vi "retrieveGoalAmount.vi"(8 "error in (no error)":errorcluster, 10 "Goal.lvclass":refnum<class "Goal.lvclass">, 11 "Account History in":refnum<class "Account History.lvclass">) -> (0 "error out":errorcluster, 2 "Amount":dbl, 3 "Account History out":refnum<class "Account History.lvclass">)   [LabVIEW 2018]
uses:
  Account History.lvclass
  Goal/Goal.lvclass
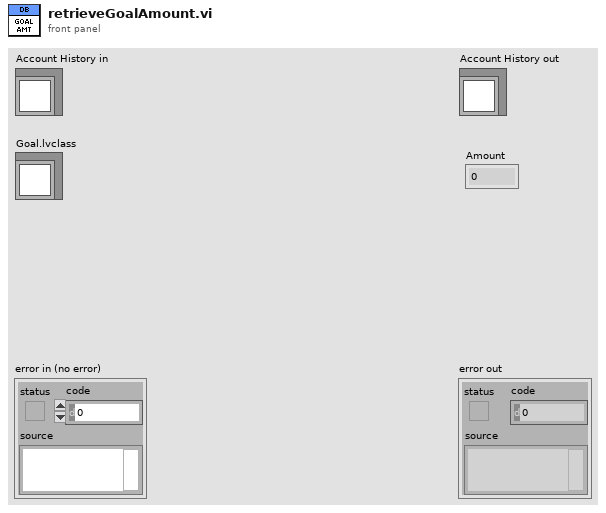
[diagram p1: front panel]
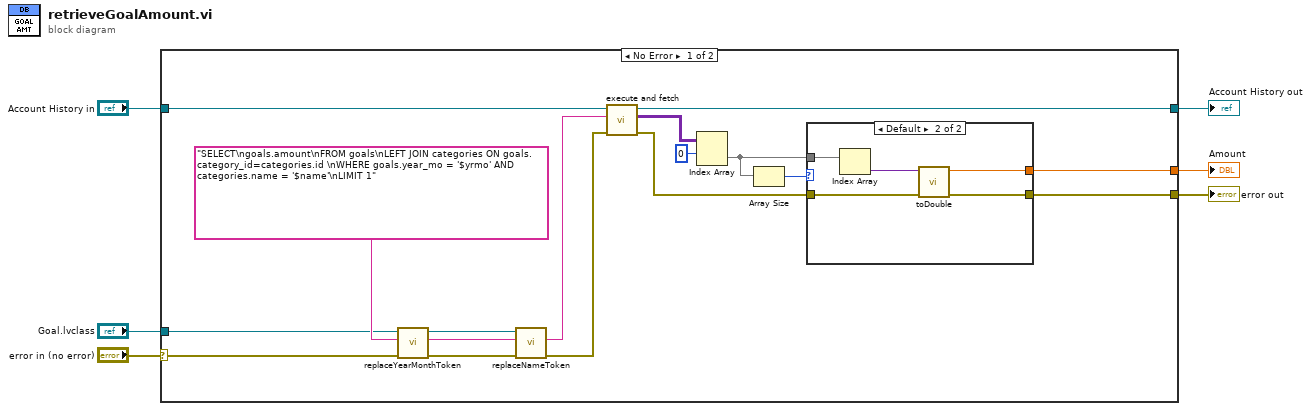
[diagram p0: block diagram]
diagram:
  n1 = case shown="No Error" "error in (no error)" {
    selector: "error in (no error)" -> [w17 w31]
    tunnel: [w21 w31] -> w5
    tunnel: [w22 w30] -> w3
    tunnel: "Account History in" -> [w23 w30]
    tunnel: "Goal.lvclass" -> [w12 _]
    tunnel: [w7 _] -> w1
    frame No Error {
      n2 = call "replaceYearMonthToken.vi"("error in (no error)"=w17, "Querry In"="SELECT\ngoals.amount\nFROM goals\nLEFT JOIN categories ON goals.category_id=categories.id \nWHERE goals.year_mo = '$yrmo' AND categories.name = '$name'\nLIMIT 1", "Goal in"=w12) -> ("error out"=w16:errorcluster, "Query Out"=w14:string, "Goal out"=w13:refnum<class "Goal.lvclass">)  [unwired: 6 in]
      n3 = call "replaceNameToken.vi"("error in (no error)"=w16, "Query In"=w14, "Goal in"=w13) -> ("error out"=w18:errorcluster, "Query Out"=w19:string)  [unwired: 6 in, 1 out]
      n4 = call "execute and fetch.vi"("error in (no error)"=w18, "SQL query"=w19, "Database in"=w23) -> ("error out"=w20:errorcluster, "recordset data"=w10:variant[][], "Database out"=w22:refnum<class "Account History.lvclass">)  [unwired: 5 in, 1 out]
      n5 = Index Array(array=w10, index (row)=0) -> (element=w9:variant[])  [unwired: 1 in]
      n6 = Array Size(array=w9) -> (size(s)=w8:i32)
      n7 = case shown="Default" w8 {
        tunnel: [w24 w26] -> w21
        tunnel: w20 -> [w24 w27]
        tunnel: w9 -> [_ w29]
        tunnel: [_ w25] -> w7
        frame 0 {
        }
        frame Default {
          n8 = Index Array(array=w29) -> (element=w28:variant)  [unwired: 1 in]
          n9 = call "toDouble.vi"("error in (no error)"=w27, "Value"=w28) -> ("error out"=w26:errorcluster, "type"=w25:dbl)  [unwired: 8 in]
        }
      }
    }
    frame Error {
    }
  }
  "error out" <- w5
  "Account History out" <- w3
  "Amount" <- w1
